vi "Update Container.vi"(7 "Container":refnum<vi>, 8 "error in (no error)":errorcluster, 10 "Item":refnum<class "Generic Item.lvclass">, 11 "StoreUI":refnum<class "StoreUI.lvclass">) -> (0 "error out":errorcluster, 3 "StoreUI 2":refnum<class "StoreUI.lvclass">)   [LabVIEW 2015, in "StoreUI.lvlib" / "StoreUI.lvclass"]
uses:
  StoreUI.lvclass
  Classes/Generic Item/Generic Item.lvclass
  Classes/Welcome Item/Welcome.lvclass
  Classes/Instrument Information/Instrument.lvclass
  Classes/Settings Item/Settings.lvclass
  StoreUI.lvclass/StoreUI.ctl
  Classes/Generic Item Messages/Invoke Container Msg/Invoke Container Msg.lvclass/Invoke Container Msg.ctl
  <vilib>/ActorFramework/Message Enqueuer/Message Enqueuer.lvclass/Message Enqueuer.ctl
  Classes/Instrument Messages/Update Details Msg/Update Details Msg.lvclass/Update Details Msg.ctl
  <vilib>/ActorFramework/Message Enqueuer/Enqueue.vi
  <vilib>/ActorFramework/Message Priority Queue/Priority Enqueue.vi
  Classes/Generic Item Messages/Invoke Container Msg/Invoke Container Msg.lvclass
  Classes/Instrument Messages/Update Details Msg/Update Details Msg.lvclass
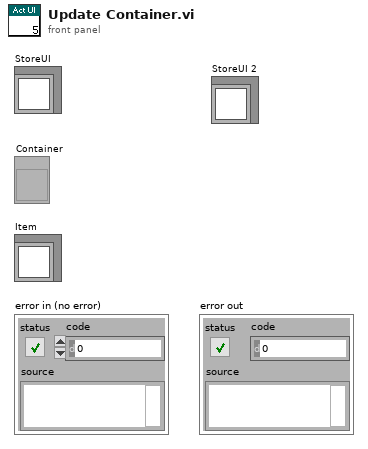
[diagram p1: front panel]
types:
  T1 = cluster{"Welcome.lvclass":refnum<class "Welcome.lvclass">, "Instrument.lvclass":refnum<class "Instrument.lvclass">, "Settings.lvclass":refnum<class "Settings.lvclass">}
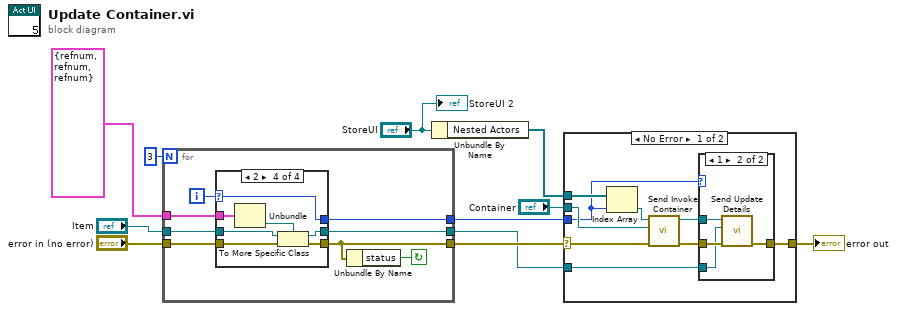
[diagram p0: block diagram]
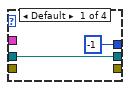
[diagram p4: hidden frame]
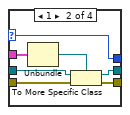
[diagram p5: hidden frame]
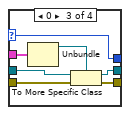
[diagram p6: hidden frame]
diagram:
  n1 = for {
    N: 3 -> [_]
    tunnel: T1 {"Welcome.lvclass"=refnum, "Instrument.lvclass"=refnum, "Settings.lvclass"=refnum} -> [w19]
    tunnel: "Item" -> [w17]
    tunnel: [w15] -> w1
    tunnel: [w14] -> w8
    tunnel: "error in (no error)" -> [w13]
    tunnel: [w12] -> w3
    i -> [w18]
    stop <- w16 continue-if-true
    n2 = case shown="2" w18 {
      selector: w18 -> [_ w23 w30 w36]
      tunnel: w19 -> [_ w28 w35 w42]
      tunnel: w17 -> [w21 w26 w34 w41]
      tunnel: [_ w25 w33 w40] -> w14
      tunnel: [w21 w24 w31 w38] -> w15
      tunnel: w13 -> [_ w22 w29 w37]
      tunnel: [-1 w23 w30 w36] -> w12
      frame Default {
      }
      frame 1 {
        n3 = Unbundle(w28) -> ("Instrument.lvclass"=w27:refnum<class "Instrument.lvclass">)  [unwired: 2 out]
        n4 = To More Specific Class(target class=w27, reference=w26, error in=w22) -> (specific class reference=w24:refnum<class "Instrument.lvclass">, error out=w25:errorcluster)
      }
      frame 0 {
        n5 = Unbundle(w35) -> ("Welcome.lvclass"=w32:refnum<class "Welcome.lvclass">)  [unwired: 2 out]
        n6 = To More Specific Class(target class=w32, reference=w34, error in=w29) -> (specific class reference=w31:refnum<class "Welcome.lvclass">, error out=w33:errorcluster)
      }
      frame 2 {
        n7 = Unbundle(w42) -> ("Settings.lvclass"=w39:refnum<class "Settings.lvclass">)  [unwired: 2 out]
        n8 = To More Specific Class(target class=w39, reference=w41, error in=w37) -> (specific class reference=w38:refnum<class "Settings.lvclass">, error out=w40:errorcluster)
      }
    }
    n9 = Unbundle By Name(w14) -> ("status"=w16:bool)
  }
  n10 = Unbundle By Name("StoreUI") -> ("Nested Actors"=w4:refnum<class "Message Enqueuer.lvclass">[])
  n11 = case shown="No Error" w8 {
    selector: w8 -> [w51 w57]
    tunnel: "Container" -> [w50 _]
    tunnel: [w45 w57] -> w5
    tunnel: w4 -> [w49 _]
    tunnel: w3 -> [w47 _]
    tunnel: w1 -> [w43 _]
    frame No Error {
      n12 = Index Array(array=w49, index=w47) -> (element=w48:refnum<class "Message Enqueuer.lvclass">)
      n13 = call "Send Invoke Container.vi"("error in (no error)"=w51, "Container"=w50, "Message Enqueuer"=w48) -> ("error out"=w46:errorcluster, "Message Enqueuer out"=w44:refnum<class "Message Enqueuer.lvclass">)  [unwired: 7 in]
      n14 = case shown="1" w47 {
        tunnel: w46 -> [w52 w56]
        tunnel: [w52 w55] -> w45
        tunnel: w44 -> [_ w54]
        tunnel: w43 -> [_ w53]
        frame Default {
        }
        frame 1 {
          n15 = call "Send Update Details.vi"("error in (no error)"=w56, "event data"=w53, "Message Enqueuer"=w54) -> ("error out"=w55:errorcluster)  [unwired: 7 in, 1 out]
        }
      }
    }
    frame Error {
    }
  }
  "error out" <- w5
  "StoreUI 2" <- "StoreUI"
